vi "doAction.vi"(8 "error in (no error)":errorcluster, 10 "ContextData":refnum<class "ContextData.lvclass">, 11 "Run in":refnum<class "Initialize References.lvclass">) -> (0 "error out":errorcluster, 2 "ContextData Out":refnum<class "ContextData.lvclass">, 3 "Run out":refnum<class "Initialize References.lvclass">)   [LabVIEW 2019, in "Initialize References.lvclass"]
uses:
  Initialize References.lvclass
  ContextData/ContextData.lvclass
  Simon_Engine/Simon_Engine.lvclass
  Messages/simonMessages/simonMessages.lvclass
  Launch UI/Launch UI.lvclass
  uiControlsMgr/uiControlsMgr.lvclass
  TextDisplay/TextDisplay Class.lvclass
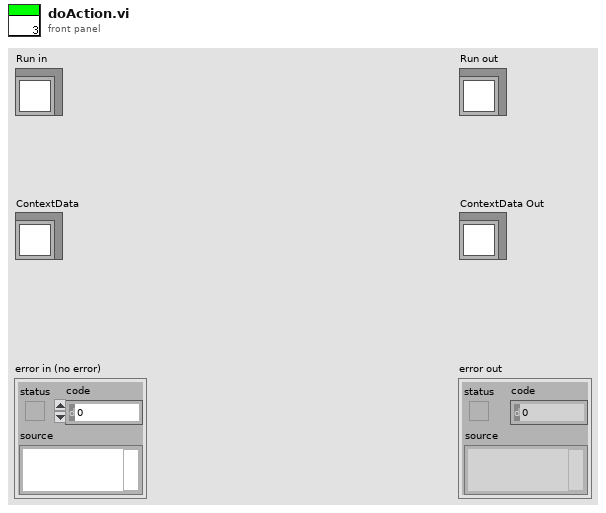
[diagram p1: front panel]
types:
  T1 = cluster{"captionsFile":string, "messageFile":string}
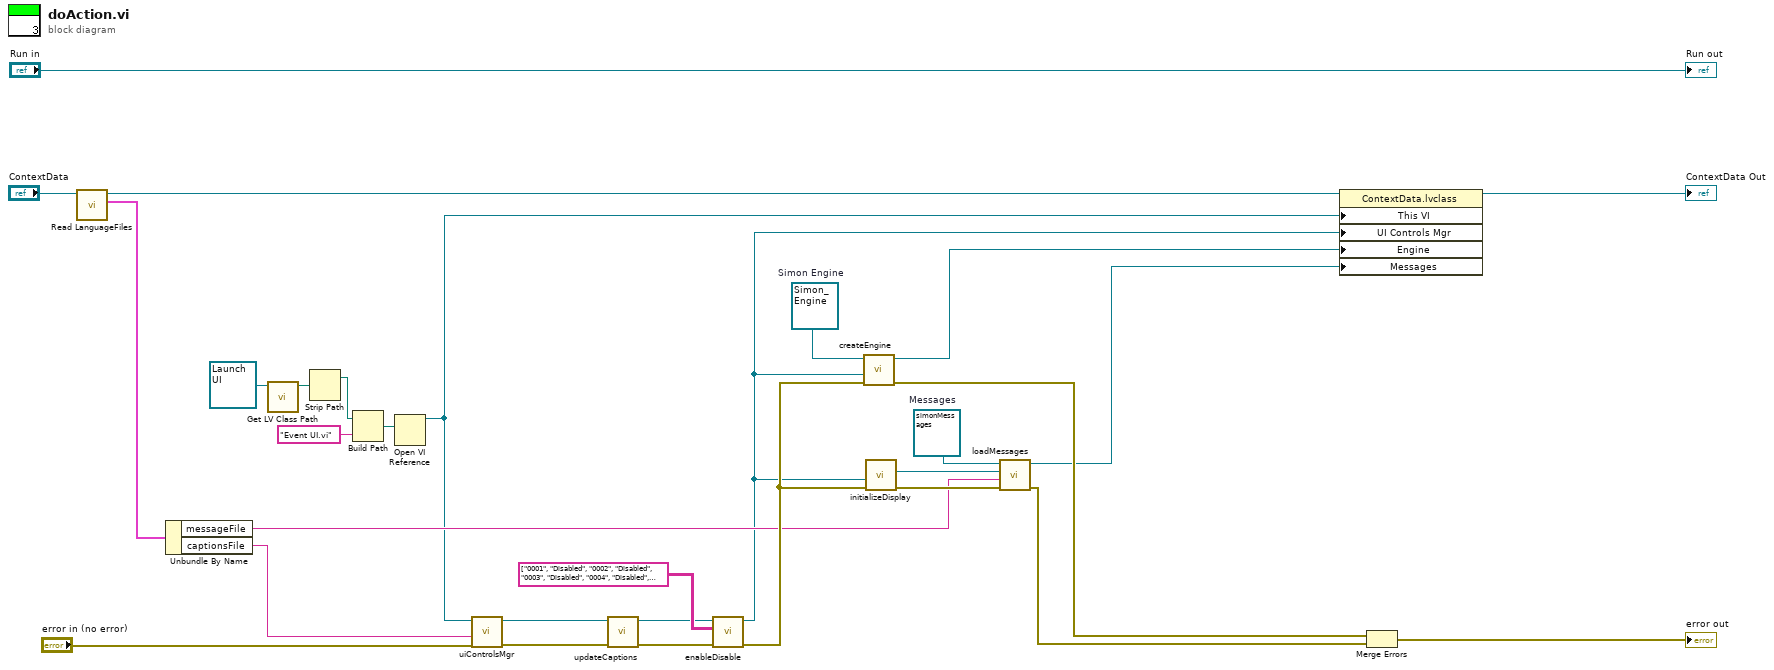
[diagram p0: block diagram]
diagram:
  w23 = refnum<class "simonMessages.lvclass"> refnum  # Messages
  w24 = refnum<class "Simon_Engine.lvclass"> refnum  # Simon Engine
  n1 = call-dynamic "Read LanguageFiles.vi"("ContextData in"="ContextData") -> ("LanguageFiles"=w26:T1, "ContextData out"=w27:refnum<class "ContextData.lvclass">)  [unwired: 8 in, 1 out]
  n2 = Unbundle By Name(w26) -> ("messageFile"=w8:string, "captionsFile"=w25:string)
  n3 = call <vilib>:"Get LV Class Path.vi"("object"=refnum<class "Launch UI.lvclass"> refnum ("Launch UI.lvclass")) -> ("class path"=w6:path)  [unwired: 9 in, 1 out]
  n4 = Strip Path(path=w6) -> (stripped path=w3:path)  [unwired: 1 out]
  n5 = Build Path(base path=w3, name or relative path="Event UI.vi") -> (appended path=w5:path)
  n6 = Open VI Reference(vi path=w5) -> (vi reference=w1:refnum<vi>)  [unwired: 5 in, 1 out]
  n7 = call "uiControlsMgr.vi"("error in (no error)"="error in (no error)", "Captions File"=w25, "VI reference"=w1) -> ("error out"=w15:errorcluster, "uiControlsMgr out"=w14:refnum<class "uiControlsMgr.lvclass">)  [unwired: 7 in]
  n8 = call "updateCaptions.vi"("error in (no error)"=w15, "uiControlsMgr in"=w14) -> ("error out"=w19:errorcluster, "uiControlsMgr out"=w18:refnum<class "uiControlsMgr.lvclass">)  [unwired: 8 in]
  n9 = call "enableDisable.vi"("error in (no error)"=w19, "Controls - Status"=string[][] [["0001", "Disabled"], ["0002", "Disabled"], ["0003", "Disabled"], ["0004", "Disabled"], ["0005", "Disabled"], ["0006", "Disabled"], ["0007", "Disabled"], ["0008", "Disabled"]], "uiControlsMgr in"=w18) -> ("error out"=w17:errorcluster, "uiControlsMgr out"=w2:refnum<class "uiControlsMgr.lvclass">)  [unwired: 7 in]
  n10 = call-dynamic "createEngine.vi"("error in (no error)"=w17, "uiControlsMgr.lvclass"=w2, "Simon_Engine in"=w24) -> ("error out"=w16:errorcluster, "Simon_Engine out"=w10:refnum<class "Simon_Engine.lvclass">)  [unwired: 7 in]
  n11 = call "initializeDisplay.vi"("error in (no error)"=w17, "uiControlsMgr.lvclass"=w2) -> ("error out"=w22:errorcluster, "TextDisplay Class out"=w21:refnum<class "TextDisplay Class.lvclass">)  [unwired: 8 in]
  n12 = call "loadMessages.vi"("error in (no error)"=w22, "FileName (without extension)"=w8, "TextDisplay"=w21, "simonMessages in"=w23) -> ("error out"=w12:errorcluster, "simonMessages out"=w9:refnum<class "simonMessages.lvclass">)  [unwired: 6 in]
  n13 = property class="ContextData.lvclass"(reference=w27, "This VI"=w1, "UI Controls Mgr"=w2, "Engine"=w10, "Messages"=w9) -> (reference out=→"ContextData Out":refnum<class "ContextData.lvclass">)  [unwired: 1 in, 1 out]
  n14 = Merge Errors(w16, w12) -> (→"error out":errorcluster)
  "Run out" <- "Run in"
